vi "Exercicio1810.vi"() -> ()   [LabVIEW 2017]
panel:
  out "Tanque 2":dbl(slide) scale=0.0..100.0
  out "Tanque 1":dbl(slide) scale=0.0..100.0
  out "Mensagem do Tanque 2":string
  out "Mensagem do Tanque 1":string
  out "LAL Tanque 2":bool caption="LAL"
  out "LAL Tanque 1":bool caption="LAL"
  out "LAH Tanque 2":bool caption="LAH"
  out "LAH Tanque 1":bool caption="LAH"
  # "Nível em %"
  # "Nível em %"
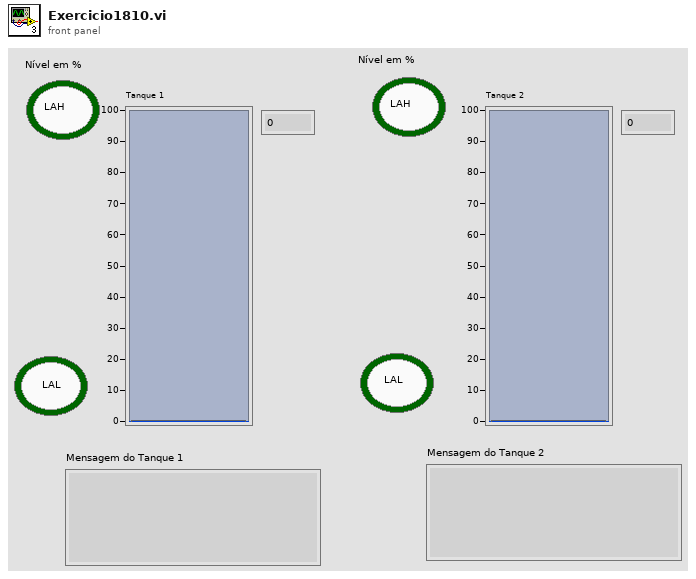
[diagram p1: front panel]
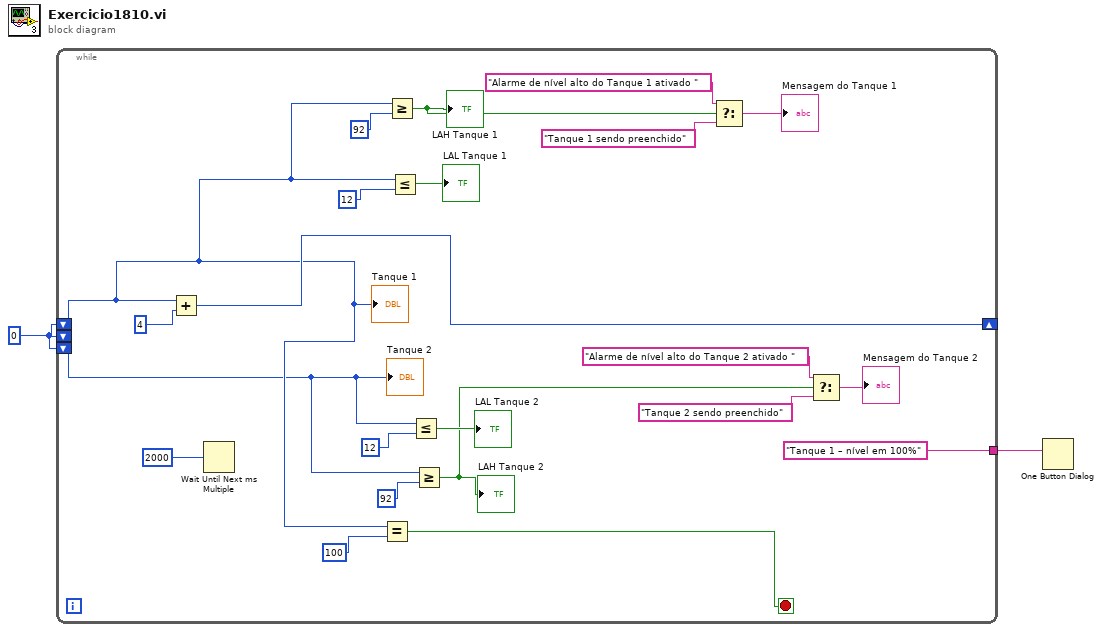
[diagram p0: block diagram]
diagram:
  w2 = 0
  n1 = while {
    shift-right: [w18] -> _
    shift-left: w2 -> [w15]
    shift-left: w2 -> [_]
    shift-left: w2 -> [w12]
    tunnel: ["Tanque 1 – nível em 100%"] -> w1
    stop <- w22 stop-if-true
    n2 = Add(x=w15, y=4) -> (x+y=w18:i32)
    n3 = Wait Until Next ms Multiple(millisecond multiple=2000) -> ()  [unwired: 1 out]
    n4 = Equal?(x=w15, y=100) -> (x = y?=w22:bool)
    n5 = Greater Or Equal?(x=w15, y=92) -> (x >= y?=w9:bool)
    "LAH Tanque 1" <- w9
    n6 = Less Or Equal?(x=w15, y=12) -> (x <= y?=→"LAL Tanque 1":bool)
    n7 = Less Or Equal?(x=w12, y=12) -> (x <= y?=→"LAL Tanque 2":bool)
    n8 = Greater Or Equal?(x=w12, y=92) -> (x >= y?=w4:bool)
    "LAH Tanque 2" <- w4
    n9 = Select(t="Alarme de nível alto do Tanque 1 ativado ", s=w9, f="Tanque 1 sendo preenchido") -> (s? t:f=→"Mensagem do Tanque 1":string)
    n10 = Select(t="Alarme de nível alto do Tanque 2 ativado ", s=w4, f="Tanque 2 sendo preenchido") -> (s? t:f=→"Mensagem do Tanque 2":string)
    "Tanque 1" <- w15
    "Tanque 2" <- w12
  }
  n11 = One Button Dialog(message=w1) -> ()  [unwired: 1 in, 1 out]
